vi "Delta_for_Equation.vi"() -> ()   [LabVIEW 2016]
uses:
  <vilib>/express/express arith-compare/Formula/XNode/ExpressFormulaBlockNode.xnode
panel:
  out "D":dbl
  in  "c":dbl
  in  "b":dbl
  in  "a":dbl
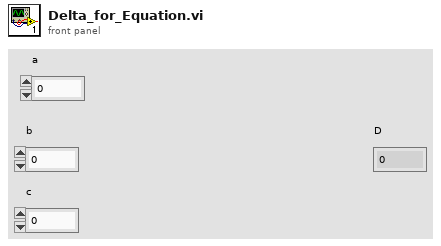
[diagram p1: front panel]
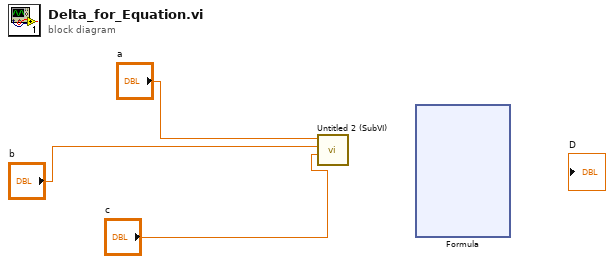
[diagram p0: block diagram]
diagram:
  n1 = call "Untitled 2 (SubVI).vi"("c"="c", "b"="b", "a"="a") -> ()  [unwired: 8 in, 1 out]
  n2 = xnode "Formula"() -> ()  [unwired: 4 in, 2 out]
